vi "rad_Select App Image Inheritance Dialog.vi"(11 "Controller Image Available?":bool) -> (0 "Cancel":bool, 1 "Disc Image":bool, 2 "Controller Image":bool, 3 "New Image":bool)   [LabVIEW 2020]
uses:
  Util/FP Control/FP Control Functions.ctl
panel:
  in  "Cancel":bool
  in  "Disc Image":bool
  in  "Controller Image":bool
  in  "New Image":bool
  # "Select image properties inheritance source..."
  # "New version of an..."
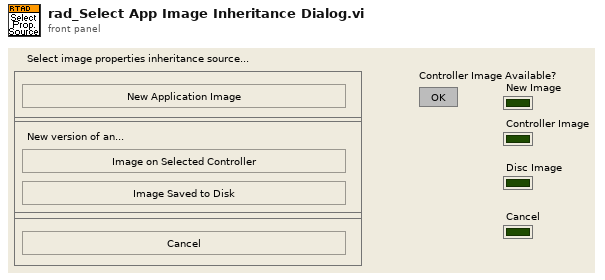
[diagram p1: front panel]
types:
  T1 = typedef "FP Control Functions.ctl" = enum16{"Open", "Close", "Bring To Front", "Center"}
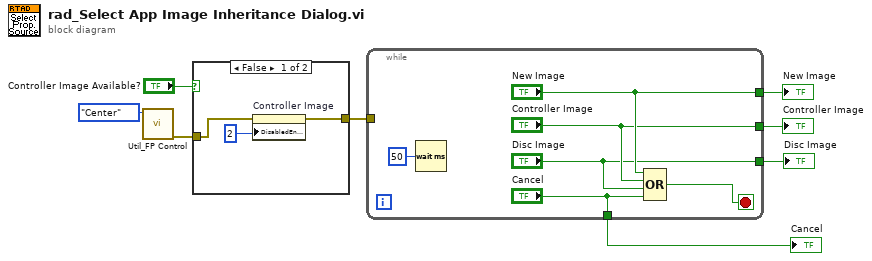
[diagram p0: block diagram]
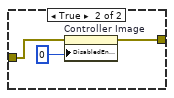
[diagram p2: hidden frame]
diagram:
  n1 = call "Util_FP Control.vi"("Function"=FP_Control_Functions."Center") -> ("error out"=w1:errorcluster)  [unwired: 1 in, 9 out]
  n2 = case shown="False" "Controller Image Available?" {
    tunnel: [w10 w13] -> w7
    tunnel: w1 -> [w9 w12]
    frame False {
      n3 = property on="Controller Image" class="Bool"(error in=w9, "DisabledEnum"=u32 2 ("milliseconds to wait")) -> (error out=w10:errorcluster)  [unwired: 1 in, 1 out]
    }
    frame True {
      n4 = property on="Controller Image" class="Bool"(error in=w12, "DisabledEnum"=u32 0 ("milliseconds to wait")) -> (error out=w13:errorcluster)  [unwired: 1 in, 1 out]
    }
  }
  n5 = while {
    tunnel: w7 -> [_]
    tunnel: ["New Image"] -> w6
    tunnel: ["Controller Image"] -> w5
    tunnel: ["Disc Image"] -> w4
    tunnel: ["Cancel"] -> w3
    stop <- w19 stop-if-true
    n6 = Wait (ms)(milliseconds to wait=u32 50) -> ()  [unwired: 1 out]
    n7 = Compound Arithmetic op=OR("New Image", "Controller Image", "Disc Image", "Cancel") -> (w19:bool)
  }
  "New Image" <- w6
  "Controller Image" <- w5
  "Disc Image" <- w4
  "Cancel" <- w3
